vi "Test Help.vi"() -> ()   [LabVIEW 2021]
uses:
  Instruments/Lockin Digitizer Driver/Lockin Digitizer Configuration.ctl
panel:
  in  "Stop Button":bool
  in  "Help Button":bool
  in  "Configuration":T1={"Post-trigger delay"=0.01, "Post-trigger duration"=0.1, "Rate"=1000000.0, "Ranges"=[10.0], "Re-name channels"=[], "Active channels"="0:1", "External\nclock"=FALSE, "Frequencies"=[], "Time\nconstant"=1.0, "Output \namplitudes"=[], "Input\nchannles"=[]} {"Output \namplitudes" format="%#_6pV"; "Time\nconstant" format="%#_6ps"; "Frequencies" format="%#_6pHz"; "Rate" format="%#_8pHz"; "Post-trigger duration" format="%#_6ps"; "Post-trigger delay" format="%#_6ps"; "Ranges" format="%#_6pV"}
  # "Digitizer config"
  # "Lock-in config"
  # "#0\n\n#1"
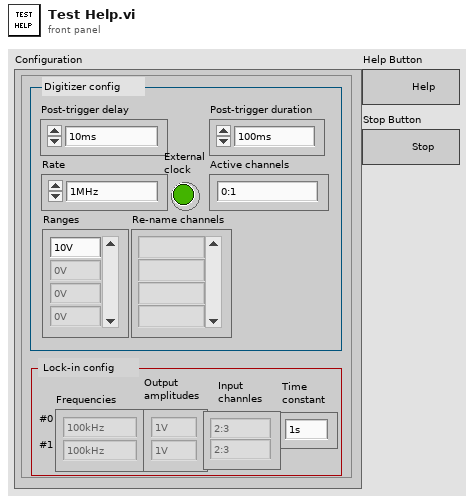
[diagram p1: front panel]
types:
  T1 = typedef "Lockin Digitizer Configuration.ctl" = cluster{"Post-trigger delay":dbl, "Post-trigger duration":dbl, "Rate":dbl, "Ranges":dbl[], "Re-name channels":string[], "Active channels":string, "External\nclock":bool, "Frequencies":dbl[], "Time\nconstant":dbl, "Output \namplitudes":dbl[], "Input\nchannles":string[]}
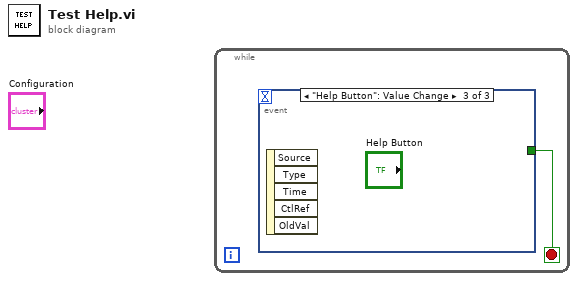
[diagram p0: block diagram]
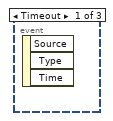
[diagram p2: hidden frame]
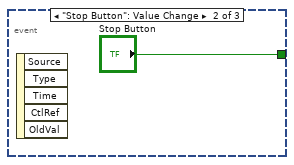
[diagram p3: hidden frame]
diagram:
  n1 = while {
    stop <- w1 stop-if-true
    n2 = event shown="[2] \"Help Button\": Value Change" {
      selector: _ -> [_ _ _]
      dyn-events: _ -> [_ _ _]
      timeout: _ -> [_ _ _]
      tunnel: [_ "Stop Button" _] -> w1
      event Timeout {
        n3 = event-data() -> ()  [unwired: 1 in, 3 out]
      }
      event "Stop Button": Value Change {
        n4 = event-data() -> ()  [unwired: 1 in, 5 out]
      }
      event "Help Button": Value Change {
        n5 = event-data() -> ()  [unwired: 1 in, 5 out]
      }
    }
  }
